vi "Test Fastest.vi"(11 "Error In":errorcluster) -> (15 "Error Out":errorcluster)   [LabVIEW 2020, in "Fastest Method Test.lvlib"]
doc: "This VI is used to validate Fastest Method"
uses:
  Fastest Method Test.lvlib
  <vilib>/addons/_JKI Toolkits/Caraya/classes/Test Suite/Define Test Suite (JUnit Report).vi
  <vilib>/SLL Drona/APIs/Stimulus/ControlValue/SetValueAuto.vi
  <vilib>/SLL Drona/APIs/Assert/AssertControlValue/Equal.vi
  <vilib>/SLL Drona/APIs/Stimulus/VI/CloseVI.vi
  <vilib>/Utility/error.llb/Error Cluster From Error Code.vi
  <vilib>/ErrorRing/Error Ring.xnode
  <vilib>/addons/_JKI Toolkits/Caraya/classes/Test Suite/Test Suite.lvclass
  <vilib>/addons/_JKI Toolkits/Caraya/classes/Test/Test.lvclass
  <vilib>/SLL Drona/Drona.lvlib
  <vilib>/SLL Drona/APIs/Stimulus/ControlValue/ControlValue.lvlib
  <vilib>/SLL Drona/APIs/Assert/AssertControlValue/AssertControlValue.lvlib
  <vilib>/Wiresmith Technology/G CLI/CLI Class/CLI.lvclass
  <vilib>/SLL Drona/APIs/Stimulus/VI/VI.lvlib
panel:
  # "FASTEST METHOD TEST"
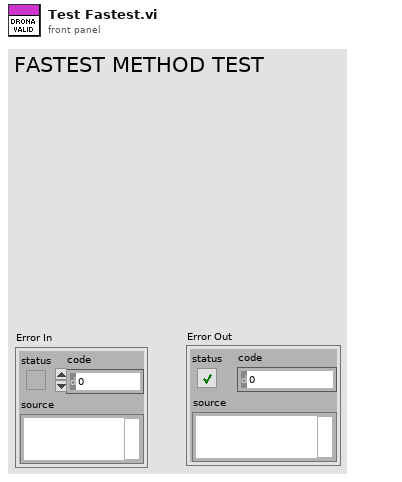
[diagram p1: front panel]
types:
  T1 = cluster{"Input X":dbl, "Fastest Method":string}[]
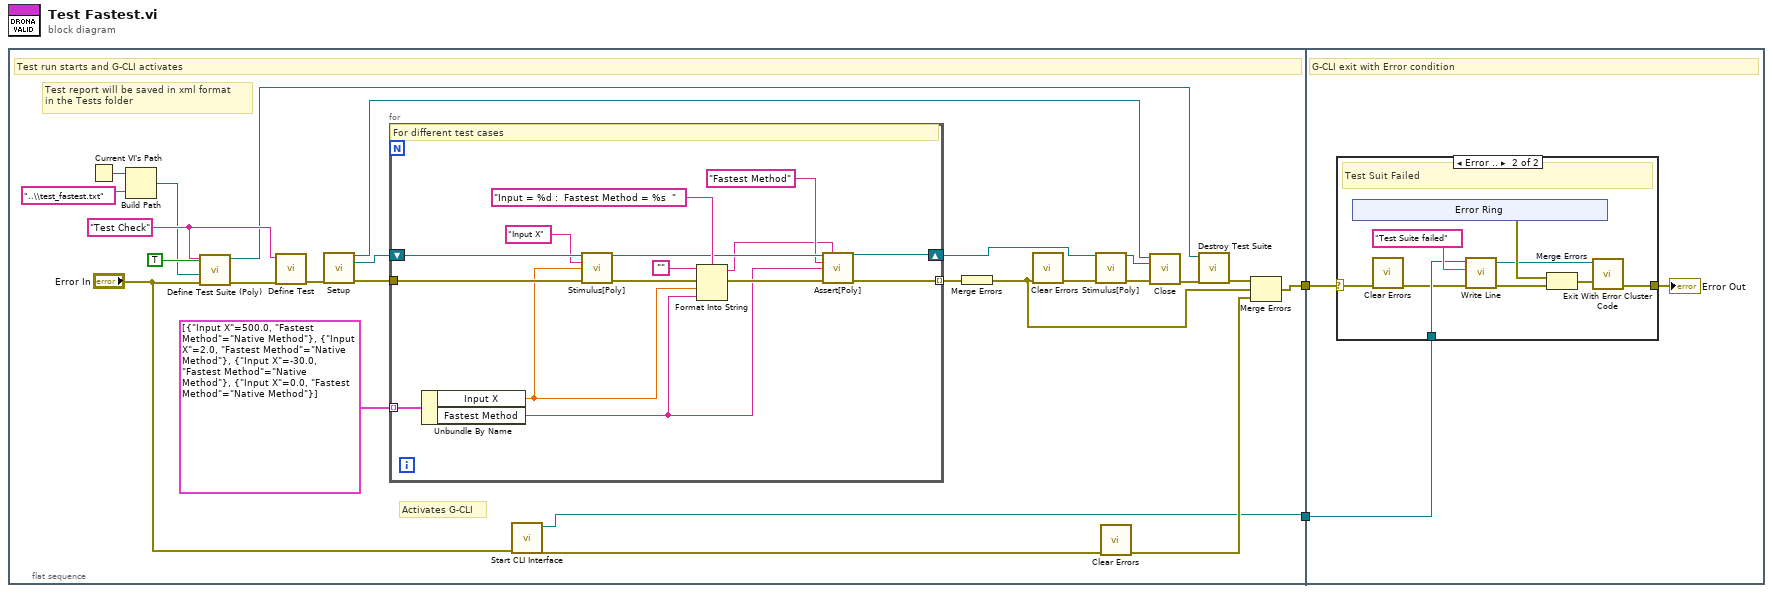
[diagram p0: block diagram]
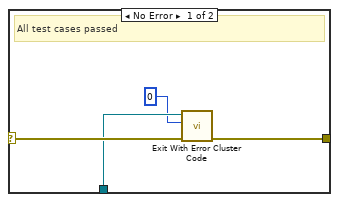
[diagram p2: hidden frame]
diagram:
  n1 = flat-sequence {
    tunnel: [w18] -> w2
    tunnel: [w8] -> w1
    tunnel: w2 -> [w45]
    tunnel: w1 -> [w44]
    frame #0 {
      w14 = "Test Check" ("Label (VI Title)")
      # "Test report will be saved in xml format\nin the Tests folder"
      # "Activates G-CLI"
      # "Test run starts and G-CLI activates"
      n2 = Current VI's Path() -> (path=w12:path)
      n3 = Build Path(base path=w12, name or relative path="..\\test_fastest.txt") -> (appended path=w10:path)
      n4 = call-poly <vilib>:"Define Test Suite (Poly).vi"("error in (no error)"="Error In", "Report Path"=w10, "Interactive"=TRUE, "Label (VI Title)"=w14) -> ("error out"=w16:errorcluster, "Test Suite"=w5:refnum<class "Test Suite.lvclass">)  [unwired: 5 in, 1 out]
      n5 = call <vilib>:"Define Test.vi"("error in (no error)"=w16, "Label (VI Title)"=w14) -> ("error out"=w27:errorcluster)  [unwired: 8 in, 1 out]
      n6 = call <vilib>:"Setup.vi"("error in"=w27) -> ("Application Ref"=w19:refnum<vi>, "VI Reference Out"=w24:refnum<vi>, "error out"=w26:errorcluster)  [unwired: 12 in]
      n7 = for {
        tunnel: w26 -> [w42]
        tunnel: T1 [{"Input X"=500.0, "Fastest Method"="Native Method"}, {"Input X"=2.0, "Fastest Method"="Native Method"}, {"Input X"=-30.0, "Fastest Method"="Native Method"}, {"Input X"=0.0, "Fastest Method"="Native Method"}] -> [w41] mode=indexing
        shift-right: [w29] -> w22
        shift-left: w24 -> [w40]
        tunnel: [w30] -> w23 mode=indexing
        # "For different test cases"
        n8 = Unbundle By Name(w41) -> ("Input X"=w35:dbl, "Fastest Method"=w31:string)
        n9 = call-poly <vilib>:"Stimulus[Poly].vi"("VI Reference In"=w40, "Control Path"="Input X", "Value (Signaling)"=w35, "error in"=w42) -> ("VI Reference Out"=w33:refnum<vi>, "error out"=w38:errorcluster)  [unwired: 10 in]
        n10 = Format Into String(format string="Input = %d :  Fastest Method = %s  ", initial string="", error in=w38, w35, w31) -> (resulting string=w28:string, error out=w34:errorcluster)
        n11 = call-poly <vilib>:"Assert[Poly].vi"("VI Reference In"=w33, "Test Label"=w28, "Control Path"="Fastest Method", "Control Value"=w31, "Error In"=w34) -> ("VI Reference Out"=w29:refnum<vi>, "Error Out"=w30:errorcluster)  [unwired: 9 in]
      }
      n12 = call <vilib>:"Start CLI Interface.vi"("error in (no error)"="Error In") -> ("error out"=w9:errorcluster, "CLI out"=w8:refnum<class "CLI.lvclass">)  [unwired: 7 in, 2 out]
      n13 = Merge Errors(w23) -> (w3:errorcluster)
      n14 = call <vilib>:"Clear Errors.vi"("error in (no error)"=w3) -> ("error out"=w4:errorcluster)  [unwired: 5 in, 1 out]
      n15 = call-poly <vilib>:"Stimulus[Poly].vi"("VI Reference In"=w22, "error in"=w4) -> ("VI Reference Out"=w20:refnum<vi>, "error out"=w21:errorcluster)  [unwired: 12 in]
      n16 = call <vilib>:"Clear Errors.vi"("error in (no error)"=w9) -> ("error out"=w17:errorcluster)  [unwired: 5 in, 1 out]
      n17 = call <vilib>:"Close.vi"("Application Ref"=w19, "VI Reference"=w20, "error in"=w21) -> ("error out"=w7:errorcluster)  [unwired: 12 in]
      n18 = call-dynamic "Destroy Test Suite.vi"("error in (no error)"=w7, "Test Suite in"=w5) -> ("error out"=w6:errorcluster)  [unwired: 8 in, 1 out]
      n19 = Merge Errors(w6, w3, w17) -> (w18:errorcluster)
    }
    frame #1 {
      # "G-CLI exit with Error condition"
      n20 = case shown="Error .." w45 {
        selector: w45 -> [w49 w53]
        tunnel: w44 -> [w48 w51]
        tunnel: [w46 w58] -> w43
        frame No Error {
          # "All test cases passed"
          n21 = call <vilib>:"Exit With Error Cluster Code.vi"("error in (no error)"=w49, "No Error Code (0)"=0, "CLI in"=w48) -> ("error out"=w46:errorcluster)  [unwired: 8 in]
        }
        frame Error {
          # "Test Suit Failed"
          n22 = xnode "Error Ring"() -> ("error out"=w55:errorcluster)
          n23 = call <vilib>:"Clear Errors.vi"("error in (no error)"=w53) -> ("error out"=w50:errorcluster)  [unwired: 5 in, 1 out]
          n24 = call <vilib>:"Write Line.vi"("error in (no error)"=w50, "Text to Write"="Test Suite failed", "CLI in"=w51) -> ("error out"=w54:errorcluster, "CLI out"=w52:refnum<class "CLI.lvclass">)  [unwired: 7 in]
          n25 = Merge Errors(w55, w54) -> (w56:errorcluster)
          n26 = call <vilib>:"Exit With Error Cluster Code.vi"("error in (no error)"=w56, "CLI in"=w52) -> ("error out"=w58:errorcluster)  [unwired: 9 in]
        }
      }
      "Error Out" <- w43
    }
  }
